vi "12-03-22.vi"() -> ()   [LabVIEW 2015]
uses:
  <vilib>/userdefined/High Color/IMAQdx.ctl
  <vilib>/vision/driver/IMAQdx.llb/IMAQdx Buffer Number Mode.ctl
  <vilib>/vision/driver/IMAQdx.llb/IMAQdx Acquisition Mode.ctl
  <vilib>/vision/driver/NI_Vision_Acquisition_Software.lvlib
  <vilib>/vision/NI_Vision_Development_Module.lvlib
  <vilib>/vision/Image Controls.llb/IMAQ Image.ctl
panel:
  in  "Buffer Number Mode (Next)":T1
  in  "stop":bool
  out "Found? 2":bool
  out "Style 2":string
  out "Mass (kg): 2":dbl
  out "Tong K/lg (kg) 2":dbl
  out "Quantity 2":i32
  out "Image 4":T2(plugin-control)
  in  "Session In 2":T3
  out "Buffer Number":u32
  out "Frame Rate":dbl
  out "Style":string
  out "Mass (kg):":dbl
  out "Tong K/lg (kg)":dbl
  out "Quantity":i32
  out "Image 3":T2(plugin-control)
  out "Data":string
  out "Found?":bool
  in  "Session In":T3
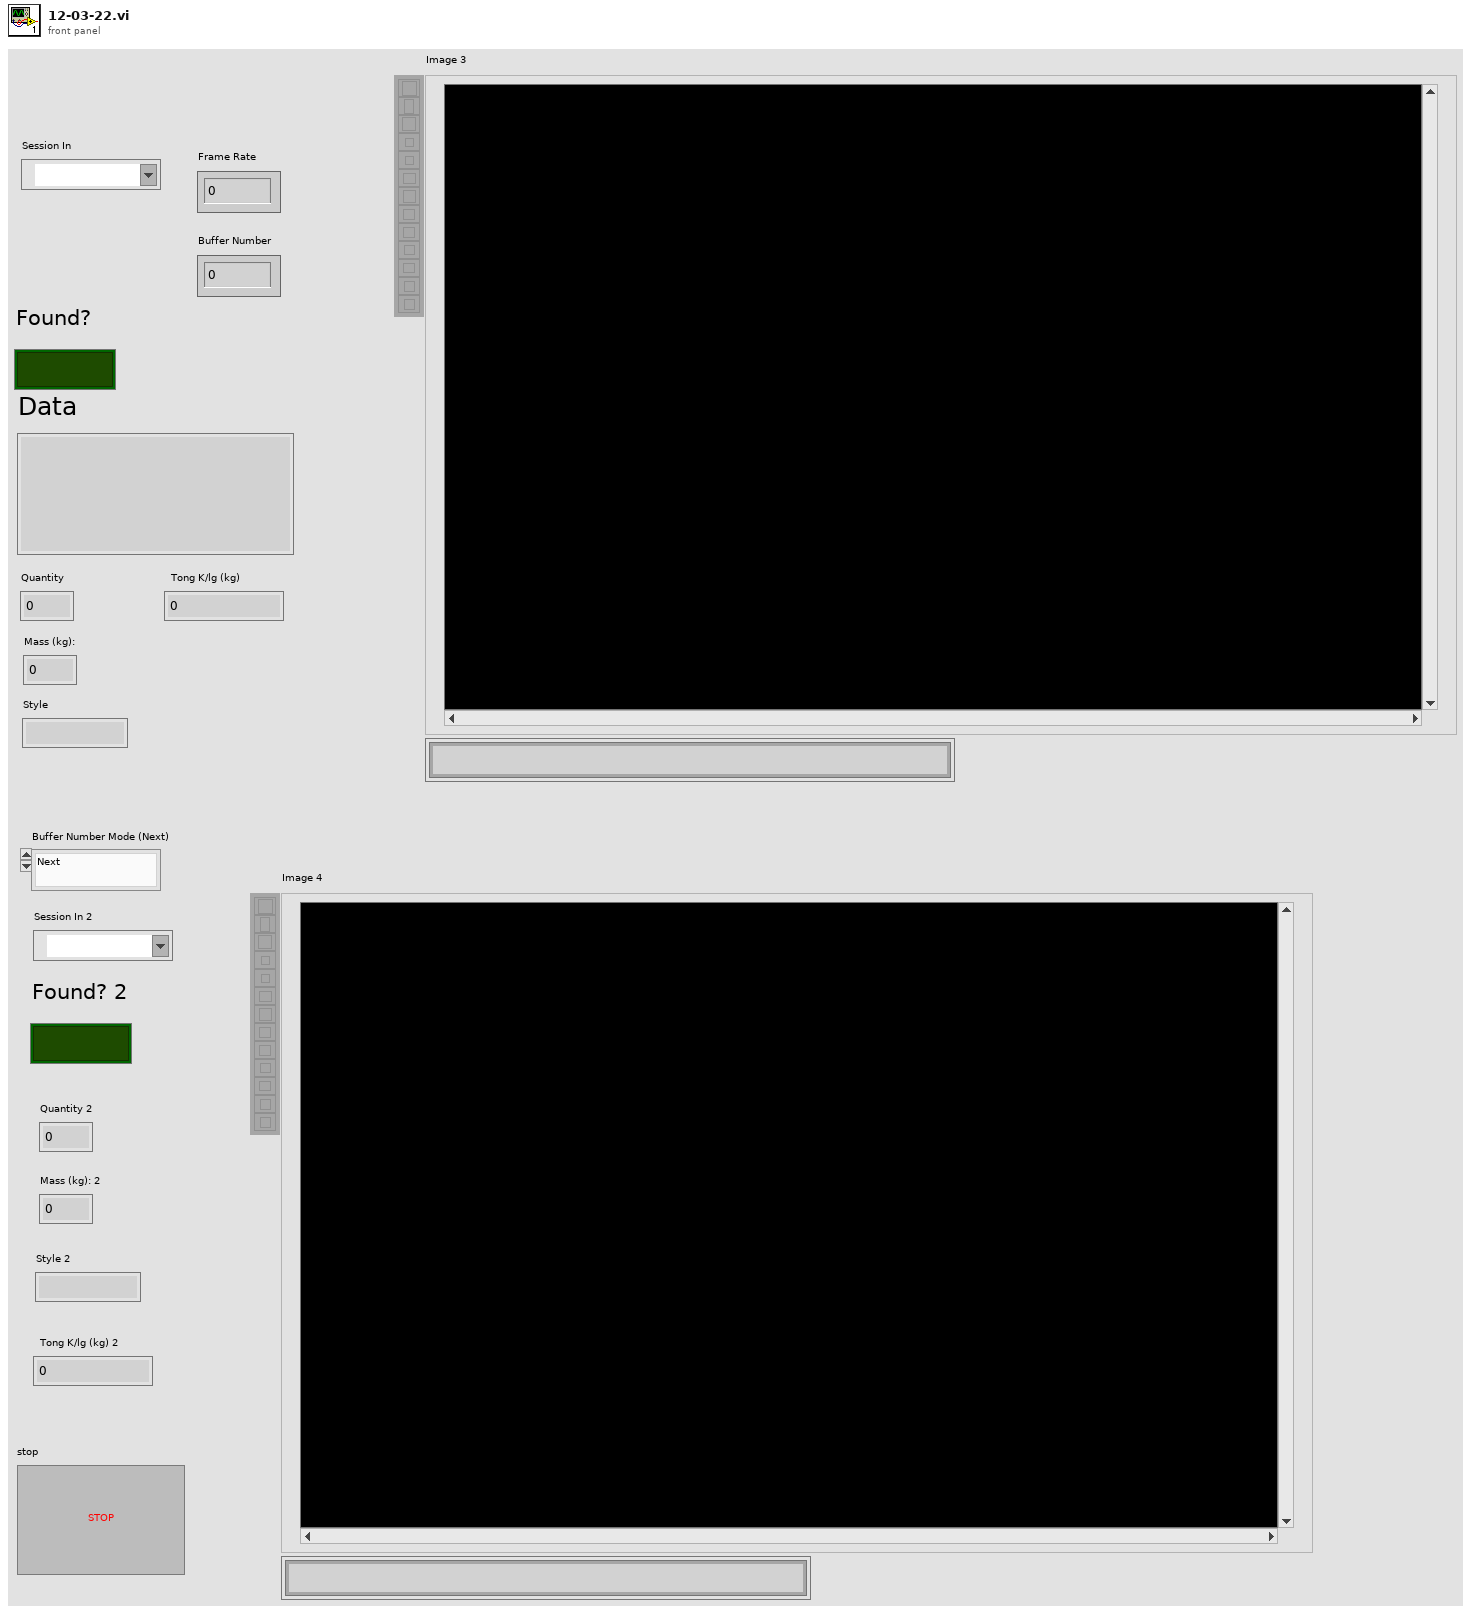
[diagram p1: front panel]
types:
  T1 = typedef "NI_Vision_Acquisition_Software.lvlib/IMAQdx Buffer Number Mode.ctl" = enum32{"Next", "Last", "Buffer Number", "Every", "Last New"}
  T2 = typedef "IMAQ Image.ctl" = refnum<image>
  T3 = typedef "IMAQdx.ctl" = refnum<k21>
  T4 = typedef "NI_Vision_Acquisition_Software.lvlib/IMAQdx Acquisition Mode.ctl" = enum32{"One Shot", "Continuous"}
  T5 = typedef "Image Type" = u32
  T6 = typedef "QR Code Report.ctl" = cluster{"Found?":bool, "Data":string, "Bounding Box":cluster{"x":sgl, "y":sgl}[], "Errors Corrected":u32, "Dimensions (Rows/Cols)":u32, "Version":u32, "QR Model":T7, "Stream Mode":T8, "Barcode Polarity":T9, "Mirrored?":bool, "Append Stream Position":u32, "Size of Append Stream":u32, "First EAN-128 ID":i32, "First Alternate Language ID":i32, "Append Stream ID":u32, "Minimum Edge Strength":u32, "Demodulation Mode":T10, "Cell Sample Size":T11, "Cell Filter Mode":T12}
  T7 = typedef "QR Code Model Type.ctl" = i32
  T8 = typedef "QR Code Stream Mode Type.ctl" = i32
  T9 = typedef "Data Matrix Polarity.ctl" = i32
  T10 = typedef "Demodulation Mode.ctl" = i32
  T11 = typedef "Cell Sample Size.ctl" = i32
  T12 = typedef "Cell Filter Mode.ctl" = i32
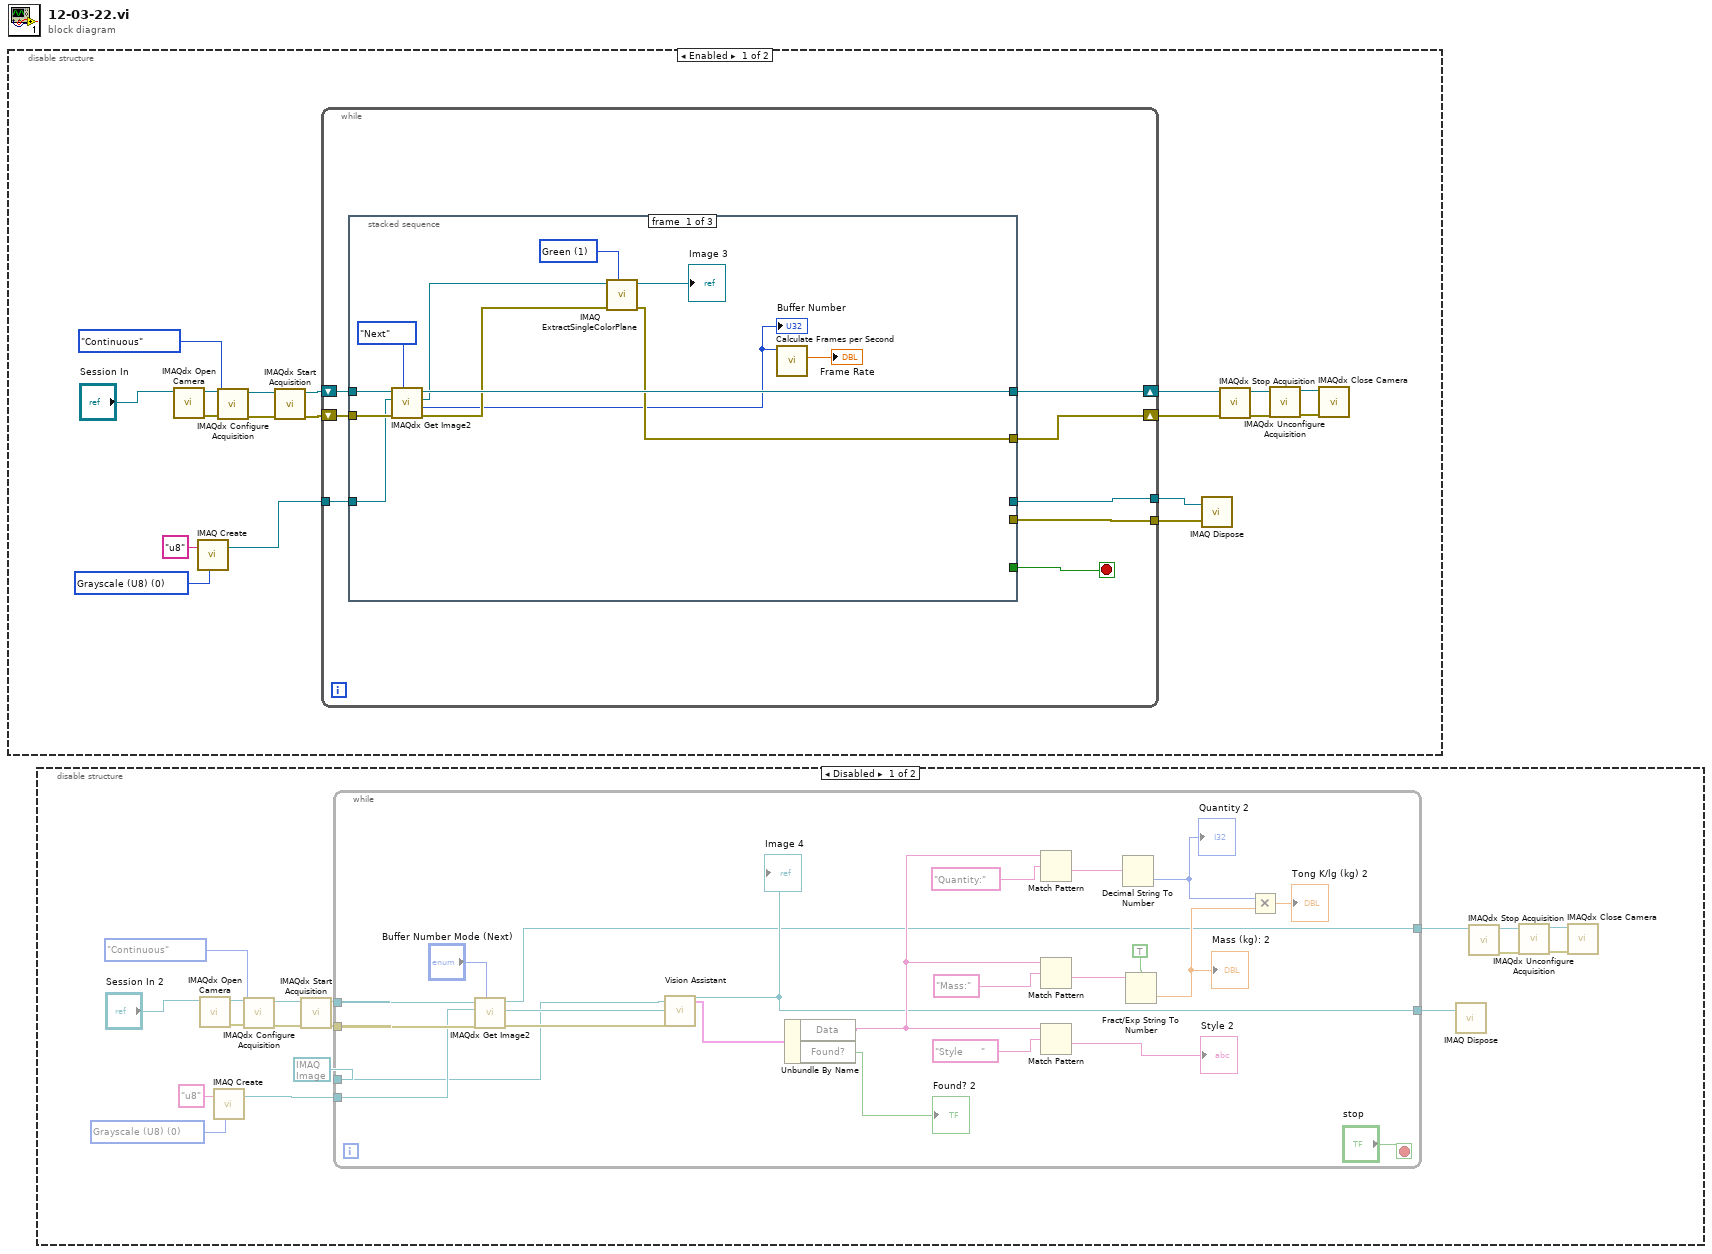
[diagram p0: block diagram]
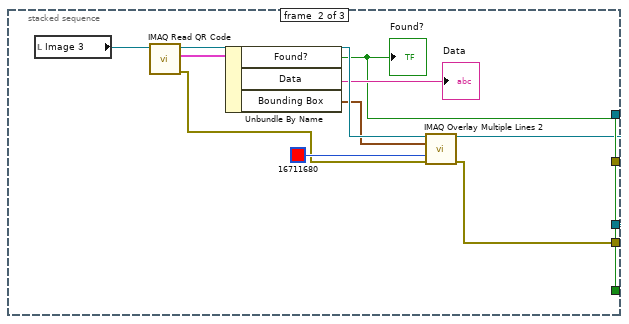
[diagram p3: hidden frame]
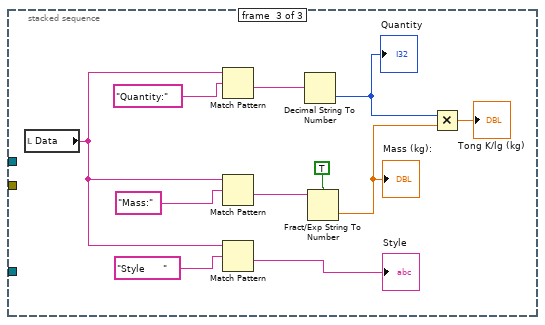
[diagram p4: hidden frame]
diagram:
  n1 = disable-structure shown="Enabled" {
    frame Enabled {
      w8 = T5 0 items=["Grayscale (U8)", "Grayscale (I16)", "Grayscale (SGL)", "Complex (CSG)", "RGB (U32)", "HSL (U32)", "RGB (U64)", "Grayscale (U16)"] ("Image Type")
      n2 = call <vilib>:"IMAQdx Open Camera.vi"("Session In"="Session In") -> ("error out"=w19:errorcluster, "Session Out"=w18:T3)  [unwired: 9 in]
      n3 = call "IMAQ Create"("Image Name"="u8", "Image Type"=w8) -> ("New Image"=w3:T2)  [unwired: 3 in, 1 out]
      n4 = call <vilib>:"IMAQdx Configure Acquisition.vi"("error in"=w19, "Continuous?"=IMAQdx_Acquisition_Mode."Continuous", "Session In"=w18) -> ("error out"=w16:errorcluster, "Session Out"=w17:T3)  [unwired: 7 in]
      n5 = call <vilib>:"IMAQdx Start Acquisition.vi"("error in"=w16, "Session In"=w17) -> ("error out"=w15:errorcluster, "Session Out"=w14:T3)  [unwired: 8 in]
      n6 = while {
        shift-right: [w23] -> w6
        shift-left: w15 -> [w27]
        shift-right: [w25] -> w7
        shift-left: w14 -> [w26]
        tunnel: w3 -> [w22]
        tunnel: [w21] -> w2
        tunnel: [w20] -> w1
        stop <- w24 stop-if-true
        n7 = stacked-sequence {
          tunnel: w27 -> [w39 _ _]
          tunnel: w26 -> [w38 _ _]
          tunnel: w22 -> [w37 _ _]
          tunnel: [w36 _ _] -> w25
          tunnel: [_ w42 _] -> w21
          tunnel: [_ w43 _] -> w24
          tunnel: [w30 _ _] -> w23
          tunnel: [_ w40 _] -> w20
          frame #0 {
            w33 = 1 items=["Red", "Green", "Blue", "Hue", "Saturation", "Luminance", "Value", "Intensity"] ("Color Plane")
            n8 = call <vilib>:"IMAQdx Get Image2.vi"("Buffer Number Mode (Next)"=IMAQdx_Buffer_Number_Mode."Next", "error in"=w39, "Image In"=w37, "Session In"=w38) -> ("error out"=w34:errorcluster, "Buffer Number Out"=w28:u32, "Image Out"=w35:T2, "Session Out"=w36:T3)  [unwired: 4 in]
            "Buffer Number" <- w28
            n9 = call "IMAQ ExtractSingleColorPlane"("Color Plane"=w33, "error in (no error)"=w34, "Image Src"=w35) -> ("error out"=w30:errorcluster, "Image Dst Out"=→"Image 3":T2)  [unwired: 7 in]
            n10 = call <vilib>:"Calculate Frames per Second.vi"("Buffer Number"=w28) -> ("Processed Frames/s"=→"Frame Rate":dbl)  [unwired: 8 in, 2 out]
          }
          frame #1 {
            n11 = local read "Image 3"() -> (w44:T2)
            n12 = call "IMAQ Read QR Code"("Image"=w44) -> ("error out"=w41:errorcluster, "QR Code Report"=w45:T6, "Image (duplicate)"=w49:T2)  [unwired: 7 in, 1 out]
            n13 = Unbundle By Name(w45) -> ("Found?"=w43:bool, "Data"=→"Data":string, "Bounding Box"=w46:cluster{"x":sgl, "y":sgl}[])
            "Found?" <- w43
            n14 = call "IMAQ Overlay Multiple Lines 2"("Image"=w49, "Line End Points"=w46, "Color"=u32 16711680, "error in (no error)"=w41) -> ("Image Out"=w42:T2, "error out"=w40:errorcluster)  [unwired: 10 in]
          }
          frame #2 {
            n15 = local read "Data"() -> (w50:string)
            n16 = Match Pattern(string=w50, regular expression="Quantity:") -> (after substring=w52:string)  [unwired: 1 in, 3 out]
            n17 = Match Pattern(string=w50, regular expression="Mass:") -> (after substring=w55:string)  [unwired: 1 in, 3 out]
            n18 = Match Pattern(string=w50, regular expression="Style      ") -> (after substring=→"Style":string)  [unwired: 1 in, 3 out]
            n19 = Decimal String To Number(string=w52) -> (number=w51:i32)  [unwired: 2 in, 1 out]
            "Quantity" <- w51
            n20 = Fract/Exp String To Number(use system decimal point (T)=TRUE, string=w55) -> (number=w58:dbl)  [unwired: 2 in, 1 out]
            "Mass (kg):" <- w58
            n21 = Multiply(x=w51, y=w58) -> (x*y=→"Tong K/lg (kg)":dbl)
          }
        }
      }
      n22 = call "IMAQ Dispose"("Image"=w2, "error in (no error)"=w1) -> ()  [unwired: 4 in, 1 out]
      n23 = call <vilib>:"IMAQdx Stop Acquisition.vi"("error in"=w6, "Session In"=w7) -> ("error out"=w10:errorcluster, "Session Out"=w11:T3)  [unwired: 8 in]
      n24 = call <vilib>:"IMAQdx Unconfigure Acquisition.vi"("error in"=w10, "Session In"=w11) -> ("error out"=w13:errorcluster, "Session Out"=w12:T3)  [unwired: 8 in]
      n25 = call <vilib>:"IMAQdx Close Camera.vi"("error in"=w13, "Session In"=w12) -> ()  [unwired: 9 in, 1 out]
    }
    frame Disabled {
    }
  }
  n26 = disable-structure shown="Disabled" {
    frame Disabled {
      w69 = T5 0 items=["Grayscale (U8)", "Grayscale (I16)", "Grayscale (SGL)", "Complex (CSG)", "RGB (U32)", "HSL (U32)", "RGB (U64)", "Grayscale (U16)"] ("Image Type")
      n27 = call <vilib>:"IMAQdx Open Camera.vi"("Session In"="Session In 2") -> ("error out"=w78:errorcluster, "Session Out"=w77:T3)  [unwired: 9 in]
      n28 = call "IMAQ Create"("Image Name"="u8", "Image Type"=w69) -> ("New Image"=w68:T2)  [unwired: 3 in, 1 out]
      n29 = call <vilib>:"IMAQdx Configure Acquisition.vi"("error in"=w78, "Continuous?"=IMAQdx_Acquisition_Mode."Continuous", "Session In"=w77) -> ("error out"=w75:errorcluster, "Session Out"=w76:T3)  [unwired: 7 in]
      n30 = call <vilib>:"IMAQdx Start Acquisition.vi"("error in"=w75, "Session In"=w76) -> ("error out"=w71:errorcluster, "Session Out"=w72:T3)  [unwired: 8 in]
      n31 = while {
        tunnel: w72 -> [w101]
        tunnel: w71 -> [w100]
        tunnel: w68 -> [w99]
        tunnel: [w84] -> w67
        tunnel: [w83] -> w62
        tunnel: T2 refnum ("Image Dst") -> [w82]
        stop <- "stop" stop-if-true
        n32 = call <vilib>:"IMAQdx Get Image2.vi"("Buffer Number Mode (Next)"="Buffer Number Mode (Next)", "error in"=w100, "Image In"=w99, "Session In"=w101) -> ("error out"=w97:errorcluster, "Image Out"=w98:T2, "Session Out"=w83:T3)  [unwired: 4 in, 1 out]
        n33 = call "Vision Assistant"("Image In"=w98, "Image Dst"=w82, "error in"=w97) -> ("Image Out"=w84:T2, "QR Barcode Report (2D Barcode Reader 1)"=w96:T6)  [unwired: 22 in, 1 out]
        "Image 4" <- w84
        n34 = Unbundle By Name(w96) -> ("Data"=w85:string, "Found?"=→"Found? 2":bool)
        n35 = Match Pattern(string=w85, regular expression="Quantity:") -> (after substring=w87:string)  [unwired: 1 in, 3 out]
        n36 = Match Pattern(string=w85, regular expression="Mass:") -> (after substring=w90:string)  [unwired: 1 in, 3 out]
        n37 = Match Pattern(string=w85, regular expression="Style      ") -> (after substring=→"Style 2":string)  [unwired: 1 in, 3 out]
        n38 = Decimal String To Number(string=w87) -> (number=w86:i32)  [unwired: 2 in, 1 out]
        "Quantity 2" <- w86
        n39 = Fract/Exp String To Number(use system decimal point (T)=TRUE, string=w90) -> (number=w93:dbl)  [unwired: 2 in, 1 out]
        "Mass (kg): 2" <- w93
        n40 = Multiply(x=w86, y=w93) -> (x*y=→"Tong K/lg (kg) 2":dbl)
      }
      n41 = call "IMAQ Dispose"("Image"=w67) -> ()  [unwired: 5 in, 1 out]
      n42 = call <vilib>:"IMAQdx Stop Acquisition.vi"("Session In"=w62) -> ("error out"=w63:errorcluster, "Session Out"=w64:T3)  [unwired: 9 in]
      n43 = call <vilib>:"IMAQdx Unconfigure Acquisition.vi"("error in"=w63, "Session In"=w64) -> ("error out"=w66:errorcluster, "Session Out"=w65:T3)  [unwired: 8 in]
      n44 = call <vilib>:"IMAQdx Close Camera.vi"("error in"=w66, "Session In"=w65) -> ()  [unwired: 9 in, 1 out]
    }
    frame Enabled {
    }
  }
